vi "Match with Submatch1 Info.vi"(8 "offset past match in":i32, 9 "regular expression":string, 10 "string":string) -> (0 "offset past whole match":i32, 1 "match found?":bool, 2 "submatch 1":T1)   [LabVIEW 2020, in "Explain Error Improved Dialog.lvlib"]
uses:
  Explain Error Improved Dialog/Explain Error Improved Dialog.lvlib
  <vilib>/regexp/Match Regular Expression.xnode
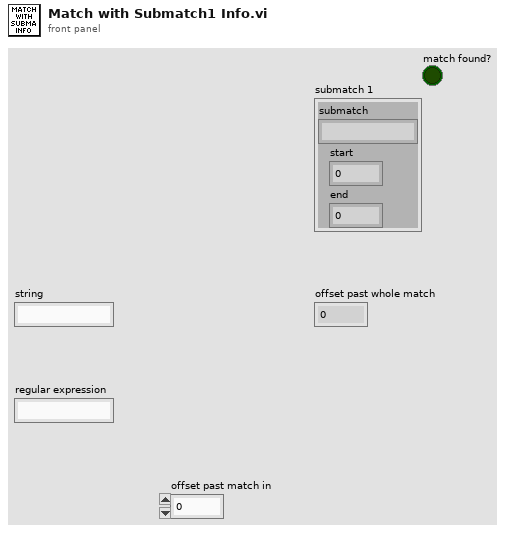
[diagram p1: front panel]
types:
  T1 = cluster{"submatch":string, "start":i32, "end":i32}
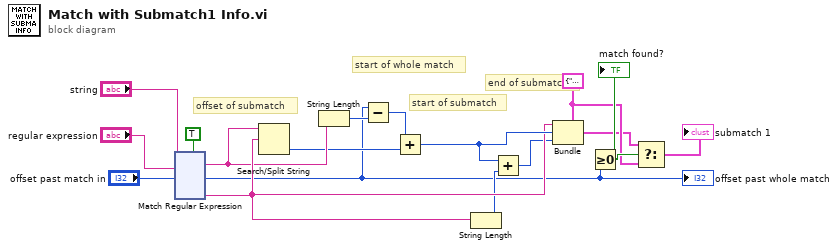
[diagram p0: block diagram]
diagram:
  w3 = T1 {"submatch"="", "start"=0, "end"=0} ("submatch")
  # "end of submatch"
  # "start of submatch"
  # "start of whole match"
  # "offset of submatch"
  n1 = xnode "Match Regular Expression"("input string"="string", "regular expression"="regular expression", "offset (0)"="offset past match in", "multiline? (F)"=TRUE) -> ("whole match"=w12:string, "offset past match"=w5:i32, "submatch 1"=w15:string)  [unwired: 2 in, 3 out]
  "offset past whole match" <- w5
  n2 = Search/Split String(string=w12, search string/char (-)=w15) -> (offset of match=w11:i32)  [unwired: 1 in, 2 out]
  n3 = String Length(string=w12) -> (length=w9:i32)
  n4 = Subtract(x=w5, y=w9) -> (x-y=w10:i32)
  n5 = Add(x=w10, y=w11) -> (x+y=w17:i32)
  n6 = String Length(string=w15) -> (length=w13:i32)
  n7 = Add(x=w17, y=w13) -> (x+y=w14:i32)
  n8 = Bundle(cluster=w3, "submatch"=w15, "start"=w17, "end"=w14) -> (w2:T1)
  n9 = Greater Or Equal To 0?(x=w5) -> (x >= 0?=w4:bool)
  "match found?" <- w4
  n10 = Select(t=w2, s=w4, f=w3) -> (s? t:f=→"submatch 1":T1)
